vi "convertPhysicalChannel.vi"(8 "error in (no error)":errorcluster, 10 "physicalChannels":string, 11 "K2602 in":refnum<class "K2602.lvclass">) -> (0 "error out":errorcluster, 2 "channel":i32[](array[numeric]), 3 "K2602 out":refnum<class "K2602.lvclass">)   [LabVIEW 2011, in "Hardware.lvlib" / "Channels.lvlib" / "K2602.lvclass"]
uses:
  K2602.lvclass
  K2602.lvclass/K2602.ctl
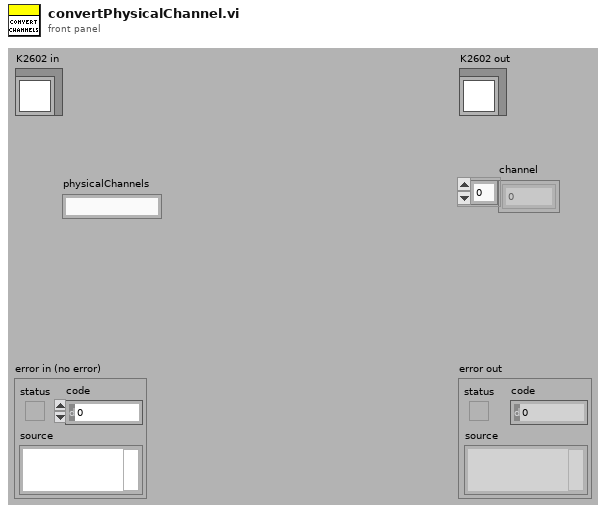
[diagram p1: front panel]
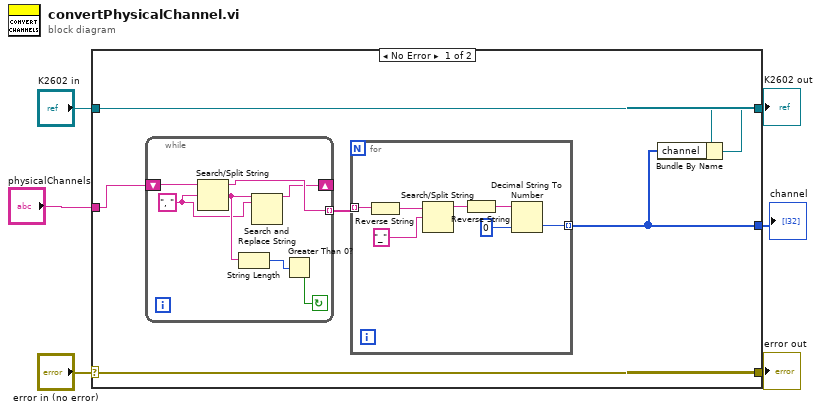
[diagram p0: block diagram]
diagram:
  n1 = case shown="No Error" "error in (no error)" {
    selector: "error in (no error)" -> [w12 w28]
    tunnel: [w12 w28] -> w5
    tunnel: [w8 w27] -> w3
    tunnel: "K2602 in" -> [w9 w27]
    tunnel: "physicalChannels" -> [w10 _]
    tunnel: [w7 _] -> w1
    frame No Error {
      n2 = while {
        shift-right: [w15] -> _
        shift-left: w10 -> [w19]
        tunnel: [w18] -> w11 mode=indexing
        stop <- w13 continue-if-true
        w16 = ", "
        n3 = Search/Split String(string=w19, search string/char (-)=w16) -> (substring before match=w18:string, match + rest of string=w17:string)  [unwired: 1 in, 1 out]
        n4 = String Length(string=w17) -> (length=w14:i32)
        n5 = Search and Replace String(input string=w17, search string=w16) -> (result string=w15:string)  [unwired: 6 in, 3 out]
        n6 = Greater Than 0?(x=w14) -> (x > 0?=w13:bool)
      }
      n7 = for {
        tunnel: w11 -> [w26] mode=indexing
        tunnel: [w21] -> w7 mode=indexing
        n8 = Reverse String(1:w26) -> (0:w25:string)
        n9 = Search/Split String(string=w25, search string/char (-)="_") -> (substring before match=w23:string)  [unwired: 1 in, 2 out]
        n10 = Reverse String(1:w23) -> (0:w22:string)
        n11 = Decimal String To Number(string=w22, default (0L)=0) -> (number=w21:i32)  [unwired: 1 in, 1 out]
      }
      n12 = Bundle By Name(cluster=w9, "channel"=w7) -> (w8:refnum<class "K2602.lvclass">)
    }
    frame Error {
    }
  }
  "error out" <- w5
  "K2602 out" <- w3
  "channel" <- w1
